vi "A34401Fetch Measurement (Fetch).vi"(8 "error in (no error)":errorcluster, 10 "Timeout (10000 ms)":u32=10000, 11 "VISA resource name":refnum<visa-resource-name>) -> (0 "error out":errorcluster, 1 "End of Data?":bool=TRUE, 2 "Measurements":dbl[](array[numeric]), 3 "VISA resource name out":refnum<visa-resource-name>)   [LabVIEW 2019, in "A34401Agilent 34401.lvlib"]
doc: "Fetches measurement from the instrument. This VI sends the \"FETCH\" command to the instrument and is to be used after \"INIT\" has been called. The VI will also wait until all data is returned before completing.\n\n<B>Note:</B>\n\nThis VI is called by <B>Fetch Measurement VI</B> in the following cases:\n(1) Model = 34401 and Trigger Source = Software\n(2) Model = 34410/34411, Trigger Source = Software, and Math = On"
uses:
  A34401Agilent 34401.lvlib
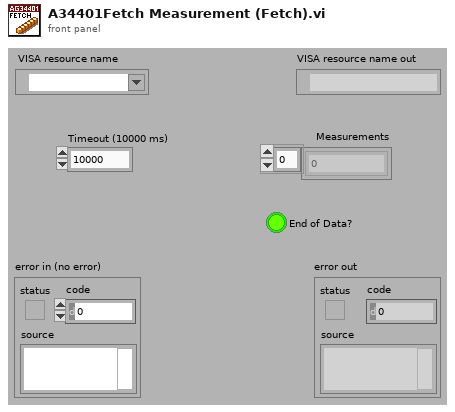
[diagram p1: front panel]
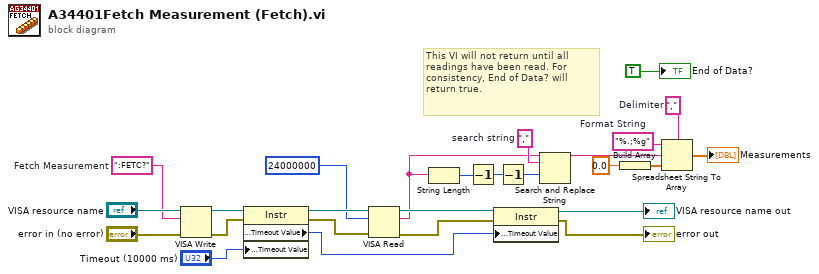
[diagram p0: block diagram]
diagram:
  w10 = ","  # search string
  w13 = ","  # Delimiter
  w14 = "%.;%g"  # Format String
  w24 = ":FETC?"  # Fetch Measurement
  # "This VI will not return until all readings have been read. For consistency, End of Data? will return true."
  n1 = VISA Write(VISA resource name="VISA resource name", write buffer=w24, error in (no error)="error in (no error)") -> (VISA resource name out=w23:refnum<visa-resource-name>, error out=w22:errorcluster)  [unwired: 1 out]
  n2 = property on="Property Node" class="Instr"(reference=w23, error in=w22, "General Settings:Timeout Value"="Timeout (10000 ms)") -> (reference out=w21:refnum<visa-resource-name>, error out=w20:errorcluster, "General Settings:Timeout Value"=w16:u32)
  n3 = VISA Read(VISA resource name=w21, byte count=u32 24000000, error in (no error)=w20) -> (VISA resource name out=w18:refnum<visa-resource-name>, read buffer=w6:string, error out=w17:errorcluster)  [unwired: 1 out]
  n4 = String Length(string=w6) -> (length=w4:i32)
  n5 = Decrement(x=w4) -> (x-1=w5:i32)
  n6 = property on="Property Node" class="Instr"(reference=w18, error in=w17, "General Settings:Timeout Value"=w16) -> (reference out=→"VISA resource name out":refnum<visa-resource-name>, error out=→"error out":errorcluster)
  n7 = Decrement(x=w5) -> (x-1=w8:i32)
  n8 = Search and Replace String(input string=w6, search string=w10, offset=w8) -> (result string=w9:string)  [unwired: 5 in, 3 out]
  n9 = Build Array(0.0) -> (w11:dbl[])
  n10 = Spreadsheet String To Array(delimiter (Tab)=w13, format string=w14, spreadsheet string=w9, array type (2D Dbl)=w11) -> (array=→"Measurements":dbl[])
  "End of Data?" <- TRUE
